vi "Basic CVT.vi"() -> ()   [LabVIEW 2014]
uses:
  <vilib>/NI/Current Value Table/Type Defs/File Format.ctl
  <vilib>/NI/Current Value Table/Type Defs/Single Tag.ctl
  <vilib>/NI/Current Value Table/Type Defs/Data Types.ctl
  <vilib>/NI/Current Value Table/Type Defs/Tag Grouping set.ctl
  <vilib>/NI/Current Value Table/DataTypes/I32_Read.vi
  <vilib>/NI/Current Value Table/DataTypes/I32_Write.vi
  <vilib>/NI/Current Value Table/Type to Enum.vi
  <vilib>/NI/Current Value Table/DataTypes/I32_Type To Enum.vi
  <vilib>/NI/Current Value Table/FGVs/CVT Globals.vi
  <vilib>/NI/Current Value Table/FGVs/Tag Memory.vi
  <vilib>/NI/Current Value Table/Memory Block.vi
  <vilib>/NI/Current Value Table/DataTypes/I32_Memory Block.vi
  <vilib>/NI/Current Value Table/Current Value Table.lvlib
panel:
  out "Value":i32
  in  "Value In":i32=5
  in  "stop":bool
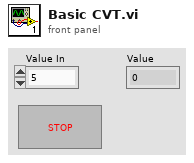
[diagram p1: front panel]
types:
  T1 = typedef "Current Value Table.lvlib/File Format.ctl" = cluster{"Tags":T2[], "Group Listings":T4[]}
  T2 = typedef "Current Value Table.lvlib/Single Tag.ctl" = cluster{"Data Type":T3, "Name":string, "Value":string, "Description":string}
  T3 = typedef "Current Value Table.lvlib/Data Types.ctl" = enum16{"Double", "Single", "I64", "I32", "I16", "I8", "U64", "U32", "U16", "U8", "String", "Boolean", "Array of U8", "Array of U16", "Array of U32", "Array of U64", "Array of I64", "Array of I32", "Array of I16", "Array of I8", "Array of Double", "Array of Single", "Array of Boolean", "Array of String"}
  T4 = typedef "Current Value Table.lvlib/Tag Grouping set.ctl" = cluster{"Group":string, "Tag Names":string[]}
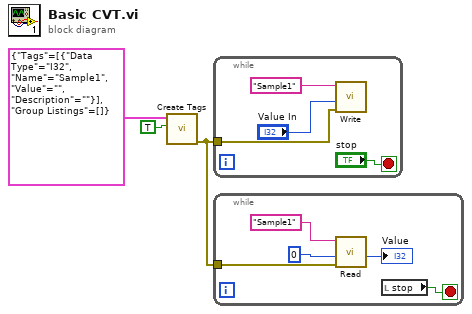
[diagram p0: block diagram]
diagram:
  n1 = call <vilib>:"Create Tags.vi"("Clear Table? (F)"=TRUE, "CVT Tags to Create"=T1 {"Tags"=[{"Data Type"=enum."I32", "Name"="Sample1", "Value"="", "Description"=""}], "Group Listings"=[]}) -> ("error out"=w1:errorcluster)  [unwired: 9 in]
  n2 = while {
    tunnel: w1 -> [w4]
    stop <- "stop" stop-if-true
    n3 = call-poly <vilib>:"Write.vi"("error in (no error)"=w4, "Value"="Value In", "Tag Name"="Sample1") -> ()  [unwired: 8 in, 1 out]
  }
  n4 = while {
    tunnel: w1 -> [w8]
    stop <- w12 stop-if-true
    n5 = call-poly <vilib>:"Read.vi"("error in (no error)"=w8, "Default"=0, "Tag Name"="Sample1") -> ("Value"=→"Value":i32)  [unwired: 7 in, 1 out]
    n6 = local read "stop"() -> (w12:bool)
  }
